vi "MergeMatchPoly.vi"(10 "Poly2D_2":T1, 11 "Poly2D_1":T1) -> (2 "Matched":bool, 3 "Poly2D":T1)   [LabVIEW 2014]
uses:
  TypeDefs/Poly2D.ctl
  TypeDefs/Point2D.ctl
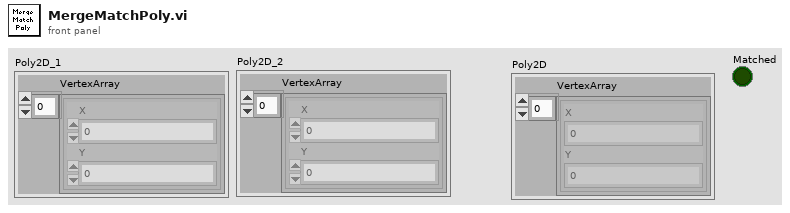
[diagram p1: front panel]
types:
  T1 = typedef "Poly2D.ctl" = cluster{"VertexArray":T2[]}
  T2 = typedef "Point2D.ctl" = cluster{"X":sgl, "Y":sgl}
  T3 = enum16{"V1V1", "V1V2", "V2V1", "V2V2", "NoMatch"}
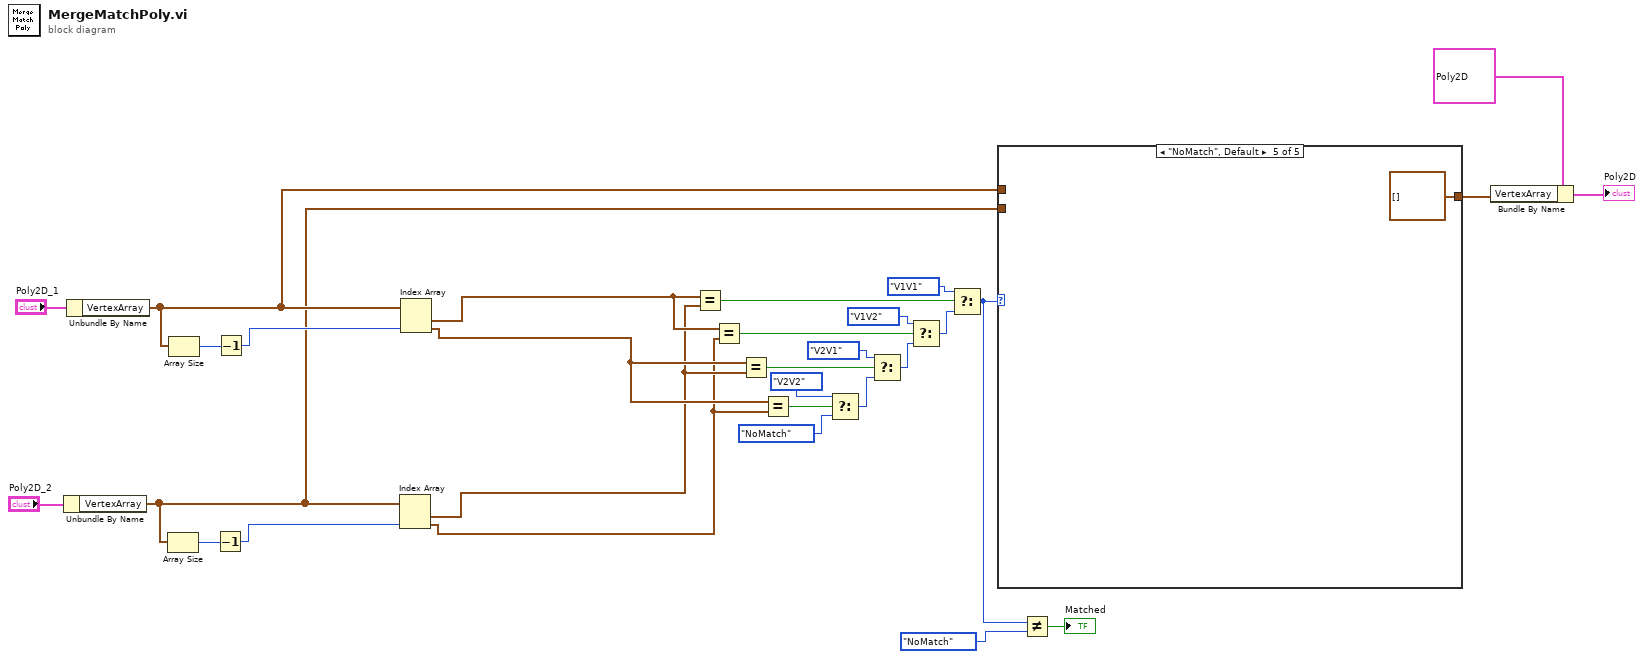
[diagram p0: block diagram]
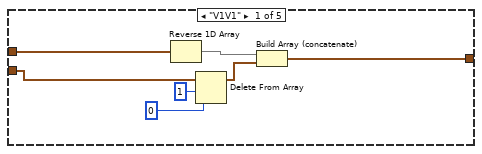
[diagram p2: hidden frame]
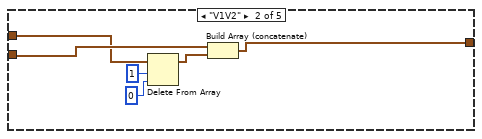
[diagram p3: hidden frame]
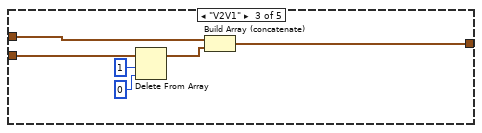
[diagram p4: hidden frame]
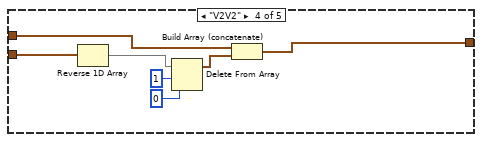
[diagram p5: hidden frame]
diagram:
  n1 = Unbundle By Name("Poly2D_2") -> ("VertexArray"=w4:T2[])
  n2 = Unbundle By Name("Poly2D_1") -> ("VertexArray"=w6:T2[])
  n3 = Array Size(array=w4) -> (size(s)=w27:i32)
  n4 = Array Size(array=w6) -> (size(s)=w30:i32)
  n5 = Decrement(x=w27) -> (x-1=w28:i32)
  n6 = Decrement(x=w30) -> (x-1=w29:i32)
  n7 = Index Array(array=w4, index #2=w28) -> (element #1=w9:T2, element #2=w8:T2)  [unwired: 1 in]
  n8 = Index Array(array=w6, index #2=w29) -> (element #1=w11:T2, element #2=w10:T2)  [unwired: 1 in]
  n9 = Equal?(x=w11, y=w9) -> (x = y?=w26:bool)
  n10 = Equal?(x=w11, y=w8) -> (x = y?=w24:bool)
  n11 = Equal?(x=w10, y=w9) -> (x = y?=w23:bool)
  n12 = Equal?(x=w10, y=w8) -> (x = y?=w21:bool)
  n13 = Select(t=T3."V2V2" ("f"), s=w21, f=T3."NoMatch") -> (s? t:f=w20:T3)
  n14 = Select(t=T3."V2V1" ("f"), s=w23, f=w20) -> (s? t:f=w22:T3)
  n15 = Select(t=T3."V1V2" ("f"), s=w24, f=w22) -> (s? t:f=w25:T3)
  n16 = Select(t=T3."V1V1" ("f"), s=w26, f=w25) -> (s? t:f=w14:T3)
  n17 = case shown="\"NoMatch\", Default" w14 {
    tunnel: w6 -> [w37 w41 w49 w55 _]
    tunnel: w4 -> [w33 w42 w47 w56 _]
    tunnel: [w35 w43 w48 w54 T2[] []] -> w2
    frame "V1V1" {
      n18 = Reverse 1D Array(array=w37) -> (reversed array=w36:T2[])
      n19 = Delete From Array(array=w33, length=1, index=0) -> (array with subset deleted=w32:T2[])  [unwired: 1 out]
      n20 = Build Array (concatenate)(w36, w32) -> (w35:T2[])
    }
    frame "V1V2" {
      n21 = Delete From Array(array=w41, length=1, index=0) -> (array with subset deleted=w38:T2[])  [unwired: 1 out]
      n22 = Build Array (concatenate)(w42, w38) -> (w43:T2[])
    }
    frame "V2V1" {
      n23 = Delete From Array(array=w47, length=1, index=0) -> (array with subset deleted=w44:T2[])  [unwired: 1 out]
      n24 = Build Array (concatenate)(w49, w44) -> (w48:T2[])
    }
    frame "V2V2" {
      n25 = Reverse 1D Array(array=w56) -> (reversed array=w53:T2[])
      n26 = Delete From Array(array=w53, length=1, index=0) -> (array with subset deleted=w52:T2[])  [unwired: 1 out]
      n27 = Build Array (concatenate)(w55, w52) -> (w54:T2[])
    }
    frame "NoMatch", Default {
    }
  }
  n28 = Not Equal?(x=w14, y=T3."NoMatch") -> (x != y?=→"Matched":bool)
  n29 = Bundle By Name(cluster=T1 {"VertexArray"=[{"X"=8.830601, "Y"=7.172068}, {"X"=9.048535, "Y"=7.0468507}, {"X"=7.186762, "Y"=7.89218}, {"X"=7.186762, "Y"=7.89218}, {"X"=7.7402935, "Y"=7.713683}, {"X"=8.830601, "Y"=7.172068}, {"X"=8.385021, "Y"=7.4258633}, {"X"=7.7402935, "Y"=7.713683}, {"X"=9.932331, "Y"=6.418683}, {"X"=9.839655, "Y"=6.4924364}, {"X"=9.9016285, "Y"=6.443779}, {"X"=9.598942, "Y"=6.669884}, {"X"=9.440515, "Y"=6.776763}, {"X"=9.048535, "Y"=7.0468507}, {"X"=8.263897, "Y"=7.4805827}, {"X"=8.113029, "Y"=7.547746}, {"X"=8.385021, "Y"=7.4258633}, {"X"=-0.8597107, "Y"=6.3534126}, {"X"=-0.7344762, "Y"=6.2797923}, {"X"=-1.3683765, "Y"=6.656569}, {"X"=-1.5755129, "Y"=6.777237}, {"X"=-1.9615697, "Y"=6.9872913}, {"X"=-0.86309165, "Y"=6.3554897}, {"X"=0.7361049, "Y"=6.279792}, {"X"=0.7496544, "Y"=6.2877717}, {"X"=0.88590366, "Y"=6.367886}, {"X"=1.1839321, "Y"=6.5489907}, {"X"=1.7457985, "Y"=6.866745}, {"X"=1.6707515, "Y"=6.8289485}, {"X"=1.5142502, "Y"=6.7378664}, {"X"=1.5142502, "Y"=6.7378664}, {"X"=1.1839321, "Y"=6.5489907}, {"X"=0.88590366, "Y"=6.367886}, {"X"=0.8825039, "Y"=6.3658695}, {"X"=-9.596155, "Y"=6.670636}, {"X"=-9.82825, "Y"=6.4999356}, {"X"=-9.82825, "Y"=6.4999356}, {"X"=-9.930481, "Y"=6.418602}, {"X"=-8.38339, "Y"=7.4258623}, {"X"=-9.046905, "Y"=7.0468526}, {"X"=-9.439066, "Y"=6.7766366}, {"X"=-7.7386646, "Y"=7.7136784}, {"X"=-8.38339, "Y"=7.4258623}, {"X"=-7.185123, "Y"=7.89218}, {"X"=-7.439444, "Y"=7.8096337}, {"X"=-7.2370896, "Y"=7.874528}, {"X"=-7.113704, "Y"=7.913477}, {"X"=-7.6962314, "Y"=7.727286}, {"X"=5.3867097, "Y"=8.087741}, {"X"=5.732113, "Y"=8.092253}, {"X"=5.9348326, "Y"=8.090443}, {"X"=6.061366, "Y"=8.076636}, {"X"=6.061366, "Y"=8.076636}, {"X"=2.5593295, "Y"=7.295466}, {"X"=2.7117634, "Y"=7.365449}, {"X"=3.1518545, "Y"=7.5595336}, {"X"=3.387326, "Y"=7.651701}, {"X"=3.6230888, "Y"=7.737315}, {"X"=3.6230888, "Y"=7.737315}, {"X"=4.127137, "Y"=7.8904243}, {"X"=4.6575503, "Y"=8.007021}, {"X"=5.21036, "Y"=8.077528}, {"X"=4.851308, "Y"=8.034141}, {"X"=3.8247945, "Y"=7.7963767}, {"X"=4.3288827, "Y"=7.9346447}, {"X"=6.589266, "Y"=8.020231}, {"X"=6.589266, "Y"=8.020231}, {"X"=7.0844173, "Y"=7.9209275}, {"X"=7.1052027, "Y"=7.9160075}, {"X"=7.1153355, "Y"=7.9134755}, {"X"=11.066484, "Y"=5.9259615}, {"X"=11.296258, "Y"=5.921032}, {"X"=10.557279, "Y"=6.071126}, {"X"=10.38447, "Y"=6.147894}, {"X"=10.217855, "Y"=6.2337523}, {"X"=10.063343, "Y"=6.3245797}, {"X"=9.958954, "Y"=6.399936}, {"X"=11.366602, "Y"=6.3154464}, {"X"=11.3581505, "Y"=6.325527}, {"X"=11.381495, "Y"=5.947889}, {"X"=11.051102, "Y"=5.927362}, {"X"=11.428065, "Y"=6.2203074}, {"X"=11.366602, "Y"=6.3154464}, {"X"=11.4614525, "Y"=6.1327662}, {"X"=11.428065, "Y"=6.2203074}, {"X"=11.465086, "Y"=6.056186}, {"X"=11.4614525, "Y"=6.1327662}, {"X"=11.438299, "Y"=5.9936595}, {"X"=11.465086, "Y"=6.056186}, {"X"=11.438299, "Y"=5.9936595}, {"X"=11.354124, "Y"=5.938431}, {"X"=11.296258, "Y"=5.921032}, {"X"=11.185439, "Y"=5.914531}, {"X"=11.114248, "Y"=5.9222054}, {"X"=10.897281, "Y"=5.9582825}, {"X"=10.843447, "Y"=5.9742303}, {"X"=10.732583, "Y"=6.0081234}, {"X"=11.066484, "Y"=5.9259615}, {"X"=10.732583, "Y"=6.0081234}, {"X"=10.719951, "Y"=6.0130906}, {"X"=10.728581, "Y"=6.0096717}, {"X"=10.450941, "Y"=6.118535}, {"X"=10.289857, "Y"=6.1987867}, {"X"=10.174761, "Y"=6.259248}, {"X"=-0.3831223, "Y"=6.131223}, {"X"=-0.06600832, "Y"=6.079455}, {"X"=0.7361049, "Y"=6.279792}, {"X"=0.49233958, "Y"=6.1676245}, {"X"=0.41289893, "Y"=6.1388397}, {"X"=0.34931928, "Y"=6.1239376}, {"X"=0.06932907, "Y"=6.079732}, {"X"=0.06932907, "Y"=6.079732}, {"X"=-0.3457704, "Y"=6.1236205}, {"X"=-0.7011162, "Y"=6.2621675}, {"X"=-0.3831223, "Y"=6.131223}, {"X"=-0.7344762, "Y"=6.2797923}, {"X"=0.020335363, "Y"=6.074264}, {"X"=-2.5576975, "Y"=7.295468}, {"X"=-2.4127276, "Y"=7.2203803}, {"X"=-2.034087, "Y"=7.027823}, {"X"=-2.5576975, "Y"=7.295468}, {"X"=-2.9499915, "Y"=7.4758196}, {"X"=-2.7095613, "Y"=7.3651953}, {"X"=-5.784939, "Y"=8.094156}, {"X"=-5.5782948, "Y"=8.096169}, {"X"=-5.3852587, "Y"=8.087761}, {"X"=-5.208071, "Y"=8.077488}, {"X"=-5.208071, "Y"=8.077488}, {"X"=-3.3850975, "Y"=7.6514883}, {"X"=-3.150348, "Y"=7.5595837}, {"X"=-3.8916922, "Y"=7.821445}, {"X"=-3.6214588, "Y"=7.73732}, {"X"=-4.6554594, "Y"=8.006941}, {"X"=-4.327599, "Y"=7.934705}, {"X"=-4.1253557, "Y"=7.890371}, {"X"=-6.50035, "Y"=8.036642}, {"X"=-6.0605617, "Y"=8.076551}, {"X"=-5.933233, "Y"=8.090459}, {"X"=-7.0827866, "Y"=7.9209275}, {"X"=-6.5884337, "Y"=8.020078}, {"X"=-7.103572, "Y"=7.916008}, {"X"=-7.103572, "Y"=7.916008}, {"X"=1.9629927, "Y"=6.9872847}, {"X"=2.0286674, "Y"=7.024026}, {"X"=2.3005672, "Y"=7.166774}, {"X"=2.4886727, "Y"=7.2611537}, {"X"=2.5593295, "Y"=7.295466}, {"X"=2.2341883, "Y"=7.1319356}, {"X"=-11.046527, "Y"=5.9253874}, {"X"=-11.183571, "Y"=5.914618}, {"X"=-11.287836, "Y"=5.9220977}, {"X"=-10.211346, "Y"=6.231735}, {"X"=-10.551163, "Y"=6.075544}, {"X"=-10.033587, "Y"=6.345599}, {"X"=-10.211346, "Y"=6.231735}, {"X"=-10.033587, "Y"=6.345599}, {"X"=-10.060636, "Y"=6.324052}, {"X"=-11.438604, "Y"=5.9953485}, {"X"=-11.465441, "Y"=6.0578756}, {"X"=-11.428589, "Y"=6.222046}, {"X"=-11.369982, "Y"=6.305766}, {"X"=-11.363838, "Y"=6.3148956}, {"X"=-11.336758, "Y"=6.3461637}, {"X"=-11.306279, "Y"=5.9260035}, {"X"=-11.38179, "Y"=5.9495883}, {"X"=-11.417481, "Y"=6.239176}, {"X"=-11.363838, "Y"=6.3148956}, {"X"=-11.428589, "Y"=6.222046}, {"X"=-11.461873, "Y"=6.134476}, {"X"=-11.46389, "Y"=6.079863}, {"X"=-11.465441, "Y"=6.0578756}, {"X"=-11.438604, "Y"=5.9953485}, {"X"=-11.38179, "Y"=5.9495883}, {"X"=-11.251305, "Y"=5.9200234}, {"X"=-11.183571, "Y"=5.914618}, {"X"=-11.046527, "Y"=5.9253874}, {"X"=-10.892313, "Y"=5.956102}, {"X"=-10.892313, "Y"=5.956102}, {"X"=-10.557951, "Y"=6.072264}, {"X"=-10.56045, "Y"=6.071302}, {"X"=-10.727159, "Y"=6.0057144}, {"X"=-10.379647, "Y"=6.146689}, {"X"=-10.379647, "Y"=6.146689}, {"X"=10.444521, "Y"=7.162137}, {"X"=10.147654, "Y"=7.396959}, {"X"=11.135348, "Y"=6.5475297}, {"X"=10.8437395, "Y"=6.8065333}, {"X"=11.135348, "Y"=6.5475297}, {"X"=7.7880063, "Y"=8.844079}, {"X"=9.709546, "Y"=7.7424564}, {"X"=9.572357, "Y"=7.8359795}, {"X"=9.48678, "Y"=7.8936634}, {"X"=9.290509, "Y"=8.026892}, {"X"=8.41312, "Y"=8.549493}, {"X"=7.7880063, "Y"=8.844079}, {"X"=10.147654, "Y"=7.396959}, {"X"=8.9828415, "Y"=8.233359}, {"X"=9.290509, "Y"=8.026892}, {"X"=8.2803135, "Y"=8.623675}, {"X"=-10.352315, "Y"=7.234274}, {"X"=-10.44289, "Y"=7.162137}, {"X"=-9.570726, "Y"=7.8359795}, {"X"=-9.707915, "Y"=7.7424564}, {"X"=-10.352315, "Y"=7.234274}, {"X"=-7.7862473, "Y"=8.8441515}, {"X"=-8.180492, "Y"=8.666639}, {"X"=-8.678174, "Y"=8.404416}, {"X"=-8.24564, "Y"=8.638364}, {"X"=-8.278681, "Y"=8.623679}, {"X"=-8.678174, "Y"=8.404416}, {"X"=-9.570726, "Y"=7.8359795}, {"X"=-9.404453, "Y"=7.9493356}, {"X"=-9.108857, "Y"=8.149092}, {"X"=-9.288878, "Y"=8.026892}, {"X"=-11.273474, "Y"=6.4113665}, {"X"=-11.126271, "Y"=6.5544534}, {"X"=-10.842109, "Y"=6.8065333}, {"X"=-10.44289, "Y"=7.162137}, {"X"=-9.838867, "Y"=7.63992}, {"X"=-9.838867, "Y"=7.63992}, {"X"=-9.608428, "Y"=7.8105674}, {"X"=2.3092422, "Y"=9.555755}, {"X"=6.897631, "Y"=9.15439}, {"X"=6.9663086, "Y"=9.135237}, {"X"=6.826199, "Y"=9.173445}, {"X"=6.826199, "Y"=9.173445}, {"X"=6.8652363, "Y"=9.162923}, {"X"=7.4247684, "Y"=8.983244}, {"X"=7.478522, "Y"=8.961372}, {"X"=6.9663086, "Y"=9.135237}, {"X"=7.0981107, "Y"=9.089703}, {"X"=-7.0928435, "Y"=9.091241}, {"X"=-7.0928435, "Y"=9.091241}, {"X"=-7.476928, "Y"=8.961346}, {"X"=-7.4378753, "Y"=8.977723}, {"X"=-2.30762, "Y"=9.555743}, {"X"=-6.9646783, "Y"=9.135236}, {"X"=-6.8925557, "Y"=9.155159}, {"X"=6.644459, "Y"=9.217671}, {"X"=4.169504, "Y"=9.464814}, {"X"=3.7893963, "Y"=9.464789}, {"X"=3.404949, "Y"=9.4514675}, {"X"=5.0040536, "Y"=9.452098}, {"X"=3.0630891, "Y"=9.468226}, {"X"=3.0630891, "Y"=9.468226}, {"X"=2.724652, "Y"=9.495395}, {"X"=2.8233345, "Y"=9.493452}, {"X"=5.3548465, "Y"=9.425313}, {"X"=5.700839, "Y"=9.381838}, {"X"=6.4296727, "Y"=9.26174}, {"X"=6.644459, "Y"=9.217671}, {"X"=6.0274963, "Y"=9.334079}, {"X"=6.0274963, "Y"=9.334079}, {"X"=5.7321496, "Y"=9.377271}, {"X"=5.4556003, "Y"=9.414961}, {"X"=5.175468, "Y"=9.441919}, {"X"=4.65047, "Y"=9.461544}, {"X"=5.0040536, "Y"=9.452098}, {"X"=4.65047, "Y"=9.461544}, {"X"=4.607755, "Y"=9.461863}, {"X"=4.169504, "Y"=9.464814}, {"X"=3.7893963, "Y"=9.464789}, {"X"=3.404949, "Y"=9.4514675}, {"X"=-2.5918474, "Y"=9.499708}, {"X"=-2.7230513, "Y"=9.495405}, {"X"=-4.4270477, "Y"=9.454551}, {"X"=-4.618484, "Y"=9.458359}, {"X"=-5.072798, "Y"=9.436931}, {"X"=-6.491574, "Y"=9.240687}, {"X"=-6.7941, "Y"=9.181162}, {"X"=-4.618484, "Y"=9.458359}, {"X"=-3.0264053, "Y"=9.4683485}, {"X"=-3.0264053, "Y"=9.4683485}, {"X"=-3.2801545, "Y"=9.449338}, {"X"=-3.2801545, "Y"=9.449338}, {"X"=-3.5855074, "Y"=9.461267}, {"X"=-3.3309553, "Y"=9.444425}, {"X"=-3.9134116, "Y"=9.468681}, {"X"=-3.6864495, "Y"=9.468745}, {"X"=-4.239195, "Y"=9.465216}, {"X"=-4.1545463, "Y"=9.471141}, {"X"=-6.2067986, "Y"=9.297449}, {"X"=-5.920551, "Y"=9.346562}, {"X"=-5.639876, "Y"=9.383647}, {"X"=-5.3612723, "Y"=9.4128685}, {"X"=-5.0972753, "Y"=9.434096}, {"X"=-4.8120456, "Y"=9.44821}, {"X"=-6.2067986, "Y"=9.297449}, {"X"=-5.920551, "Y"=9.346562}, {"X"=-5.5172114, "Y"=9.401878}, {"X"=-5.8545833, "Y"=9.354088}, {"X"=2.2132256, "Y"=9.58271}, {"X"=1.8189816, "Y"=9.648704}, {"X"=1.8189816, "Y"=9.648704}, {"X"=2.2132256, "Y"=9.58271}, {"X"=-1.6634326, "Y"=9.665585}, {"X"=-1.8177922, "Y"=9.648689}, {"X"=-2.2115984, "Y"=9.582698}, {"X"=-1.9781245, "Y"=9.618462}, {"X"=0.72814083, "Y"=12.73701}, {"X"=-0.4196546, "Y"=12.743518}, {"X"=0.0007652063, "Y"=12.753558}, {"X"=0.5166687, "Y"=12.742718}, {"X"=0.4116929, "Y"=12.74487}, {"X"=1.0176144, "Y"=12.704265}, {"X"=1.4621797, "Y"=10.655392}, {"X"=1.5545752, "Y"=9.940707}, {"X"=1.4498512, "Y"=10.855028}, {"X"=1.4578543, "Y"=10.732892}, {"X"=1.5545752, "Y"=9.940707}, {"X"=1.6384071, "Y"=9.697788}, {"X"=1.6650634, "Y"=9.665521}, {"X"=1.5937715, "Y"=9.786305}, {"X"=1.5833964, "Y"=9.82258}, {"X"=1.4787083, "Y"=10.454523}, {"X"=1.4787083, "Y"=10.454523}, {"X"=1.5225716, "Y"=10.112019}, {"X"=1.5252, "Y"=10.098917}, {"X"=1.5426022, "Y"=10.012731}, {"X"=1.5040516, "Y"=10.237594}, {"X"=1.4989743, "Y"=10.272214}, {"X"=-1.6634326, "Y"=9.665585}, {"X"=-1.6236622, "Y"=9.727999}, {"X"=-1.5983242, "Y"=9.791381}, {"X"=-1.552802, "Y"=9.935697}, {"X"=-1.5983242, "Y"=9.791381}, {"X"=-1.5869727, "Y"=9.816154}, {"X"=-1.587823, "Y"=9.813162}, {"X"=-1.5209501, "Y"=10.100272}, {"X"=-1.4973384, "Y"=10.267358}, {"X"=-1.4585742, "Y"=10.705285}, {"X"=-1.4635025, "Y"=10.629503}, {"X"=-1.4770607, "Y"=10.45756}, {"X"=-1.4482204, "Y"=10.855038}, {"X"=-1.5474311, "Y"=9.963546}, {"X"=-1.4605238, "Y"=10.667121}, {"X"=-1.4973384, "Y"=10.267358}, {"X"=-1.3789781, "Y"=11.701954}, {"X"=-1.329632, "Y"=12.03006}, {"X"=-1.4286721, "Y"=11.182402}, {"X"=-1.0699232, "Y"=12.697788}, {"X"=-1.0901189, "Y"=12.68052}, {"X"=-1.1646048, "Y"=12.571568}, {"X"=-1.2407196, "Y"=12.380032}, {"X"=-1.2720493, "Y"=12.2814455}, {"X"=-1.0159835, "Y"=12.704266}, {"X"=-1.3427985, "Y"=11.95073}, {"X"=-1.4286721, "Y"=11.182402}, {"X"=-1.4014932, "Y"=11.485938}, {"X"=-1.4188328, "Y"=11.319262}, {"X"=-1.2407196, "Y"=12.380032}, {"X"=-1.1646048, "Y"=12.571568}, {"X"=-1.0901189, "Y"=12.68052}, {"X"=1.1517563, "Y"=12.598272}, {"X"=1.04348, "Y"=12.704147}, {"X"=1.0855013, "Y"=12.679428}, {"X"=1.2149384, "Y"=12.468784}, {"X"=1.1729327, "Y"=12.554751}, {"X"=1.1517563, "Y"=12.598272}, {"X"=1.3806208, "Y"=11.686752}, {"X"=1.4204677, "Y"=11.315399}, {"X"=1.4296497, "Y"=11.192336}, {"X"=1.4498512, "Y"=10.855028}, {"X"=1.3312752, "Y"=12.016102}, {"X"=1.3806208, "Y"=11.686752}, {"X"=1.2736847, "Y"=12.293916}, {"X"=1.2751907, "Y"=12.2876835}, {"X"=1.3312752, "Y"=12.016102}, {"X"=1.2740316, "Y"=12.292477}, {"X"=1.2736847, "Y"=12.293916}, {"X"=1.1150376, "Y"=12.643135}, {"X"=-12.02701, "Y"=-8.883595}, {"X"=-11.930874, "Y"=-8.755775}, {"X"=-12.135208, "Y"=-9.147686}, {"X"=-12.100296, "Y"=-9.031299}, {"X"=-12.095111, "Y"=-9.902619}, {"X"=-12.067877, "Y"=-9.970935}, {"X"=-12.029266, "Y"=-10.067103}, {"X"=-12.029266, "Y"=-10.067103}, {"X"=-11.9856825, "Y"=-10.148499}, {"X"=-12.142309, "Y"=-9.728694}, {"X"=-12.127801, "Y"=-9.782524}, {"X"=-12.1486845, "Y"=-9.194613}, {"X"=-12.170822, "Y"=-9.369725}, {"X"=-12.1705885, "Y"=-9.389268}, {"X"=-12.168238, "Y"=-9.549478}, {"X"=-12.168238, "Y"=-9.549478}, {"X"=-11.8144655, "Y"=-8.65208}, {"X"=-11.7577095, "Y"=-8.616993}, {"X"=-11.8144655, "Y"=-8.65208}, {"X"=-12.02701, "Y"=-8.883595}, {"X"=-12.016741, "Y"=-8.869859}, {"X"=-12.135208, "Y"=-9.147686}, {"X"=-11.294352, "Y"=-10.777359}, {"X"=-11.318705, "Y"=-10.768083}, {"X"=-11.894479, "Y"=-10.297557}, {"X"=-11.864539, "Y"=-10.3413925}, {"X"=-11.542754, "Y"=-10.650674}, {"X"=-11.322815, "Y"=-10.765945}, {"X"=-11.660817, "Y"=-10.56013}, {"X"=-11.684228, "Y"=-10.5376215}, {"X"=-11.768559, "Y"=-10.456095}, {"X"=-11.768559, "Y"=-10.456095}, {"X"=-11.318705, "Y"=-10.768083}, {"X"=-11.864539, "Y"=-10.3413925}, {"X"=-11.569865, "Y"=-8.037169}, {"X"=-11.563985, "Y"=-8.070403}, {"X"=-11.552345, "Y"=-8.164364}, {"X"=-11.553843, "Y"=-8.257444}, {"X"=-11.568527, "Y"=-8.345382}, {"X"=-11.595686, "Y"=-8.425903}, {"X"=-11.632769, "Y"=-8.4943}, {"X"=-11.679456, "Y"=-8.552723}, {"X"=-11.734429, "Y"=-8.599825}, {"X"=-11.700265, "Y"=-8.574736}, {"X"=-11.650671, "Y"=-8.521496}, {"X"=-11.61017, "Y"=-8.45847}, {"X"=-11.579652, "Y"=-8.387263}, {"X"=-11.558998, "Y"=-8.305826}, {"X"=-11.550331, "Y"=-8.218866}, {"X"=-11.553987, "Y"=-8.128481}, {"X"=-11.3296585, "Y"=-13.300342}, {"X"=-11.256834, "Y"=-13.179006}, {"X"=-11.151226, "Y"=-13.057631}, {"X"=-11.16577, "Y"=-13.070827}, {"X"=-11.1825075, "Y"=-13.090706}, {"X"=-11.051586, "Y"=-12.9728775}, {"X"=-11.051586, "Y"=-12.9728775}, {"X"=-10.939525, "Y"=-12.903137}, {"X"=-10.939525, "Y"=-12.903137}, {"X"=-10.849801, "Y"=-14.563225}, {"X"=-11.164953, "Y"=-14.337027}, {"X"=-11.067114, "Y"=-14.428592}, {"X"=-11.141206, "Y"=-14.359256}, {"X"=-11.164953, "Y"=-14.337027}, {"X"=-10.933373, "Y"=-14.519123}, {"X"=-10.960547, "Y"=-14.504524}, {"X"=-11.250185, "Y"=-14.232005}, {"X"=-11.421939, "Y"=-13.710416}, {"X"=-11.408769, "Y"=-13.850409}, {"X"=-11.419471, "Y"=-13.73668}, {"X"=-11.421939, "Y"=-13.710416}, {"X"=-11.413157, "Y"=-13.569632}, {"X"=-11.382209, "Y"=-13.431717}, {"X"=-11.387743, "Y"=-13.456368}, {"X"=-11.256834, "Y"=-13.179006}, {"X"=-11.26992, "Y"=-13.200806}, {"X"=-11.321019, "Y"=-14.114156}, {"X"=-11.305685, "Y"=-14.139672}, {"X"=-11.413157, "Y"=-13.569632}, {"X"=-11.402093, "Y"=-13.876914}, {"X"=-11.374592, "Y"=-13.986052}, {"X"=-11.250185, "Y"=-14.232005}, {"X"=-11.913404, "Y"=-6.6864777}, {"X"=-11.797986, "Y"=-7.147725}, {"X"=-12.13859, "Y"=-5.825948}, {"X"=-11.913404, "Y"=-6.6864777}, {"X"=-12.225317, "Y"=-5.519531}, {"X"=-12.225317, "Y"=-5.519531}, {"X"=-11.221693, "Y"=-10.810644}, {"X"=-11.294352, "Y"=-10.777359}, {"X"=-11.030285, "Y"=-10.970268}, {"X"=-11.091174, "Y"=-10.905559}, {"X"=-11.160064, "Y"=-10.849495}, {"X"=-11.152487, "Y"=-10.854256}, {"X"=-10.860488, "Y"=-11.333081}, {"X"=-10.880931, "Y"=-11.255504}, {"X"=-10.892451, "Y"=-11.2184515}, {"X"=-10.922376, "Y"=-11.142319}, {"X"=-10.928037, "Y"=-11.131481}, {"X"=-10.928037, "Y"=-11.131481}, {"X"=-10.970161, "Y"=-11.053841}, {"X"=-11.02817, "Y"=-10.972571}, {"X"=-10.973595, "Y"=-11.048819}, {"X"=-11.028286, "Y"=-10.97244}, {"X"=-11.087512, "Y"=-10.908614}, {"X"=-10.665473, "Y"=-12.46586}, {"X"=-10.664033, "Y"=-12.508651}, {"X"=-10.673386, "Y"=-12.582449}, {"X"=-10.694738, "Y"=-12.653376}, {"X"=-10.72751, "Y"=-12.7196455}, {"X"=-10.768068, "Y"=-12.776132}, {"X"=-10.816997, "Y"=-12.825721}, {"X"=-10.902442, "Y"=-12.882612}, {"X"=-10.916191, "Y"=-12.891214}, {"X"=-10.800756, "Y"=-12.811512}, {"X"=-10.754254, "Y"=-12.759442}, {"X"=-10.716546, "Y"=-12.700924}, {"X"=-10.686941, "Y"=-12.633139}, {"X"=-10.668956, "Y"=-12.561274}, {"X"=-10.663047, "Y"=-12.487158}, {"X"=-10.665473, "Y"=-12.46586}, {"X"=-10.710455, "Y"=-14.615379}, {"X"=-10.849801, "Y"=-14.563225}, {"X"=-10.848216, "Y"=-14.563806}, {"X"=-10.7669525, "Y"=-14.595915}, {"X"=-10.30013, "Y"=-14.642541}, {"X"=-10.446137, "Y"=-14.654243}, {"X"=-10.446137, "Y"=-14.654243}, {"X"=-10.563266, "Y"=-14.646091}, {"X"=-10.469295, "Y"=-14.651767}, {"X"=-9.648653, "Y"=-14.927292}, {"X"=-9.645592, "Y"=-14.928906}, {"X"=-9.606909, "Y"=-14.948134}, {"X"=-9.606909, "Y"=-14.948134}, {"X"=-9.846963, "Y"=-14.788051}, {"X"=-9.851051, "Y"=-14.785206}, {"X"=-9.854066, "Y"=-14.783052}, {"X"=-9.772256, "Y"=-14.849932}, {"X"=-9.772256, "Y"=-14.849932}, {"X"=-9.739692, "Y"=-14.872915}, {"X"=-9.722611, "Y"=-14.884181}, {"X"=-9.722611, "Y"=-14.884181}, {"X"=-9.686776, "Y"=-14.906165}, {"X"=-12.650918, "Y"=-3.9329345}, {"X"=-12.648346, "Y"=-3.8170426}, {"X"=-12.631214, "Y"=-3.735219}, {"X"=-12.623239, "Y"=-3.7092106}, {"X"=-12.623239, "Y"=-3.7092106}, {"X"=-12.62978, "Y"=-4.049288}, {"X"=-12.650918, "Y"=-3.9329345}, {"X"=-12.57752, "Y"=-3.6137216}, {"X"=-12.57752, "Y"=-3.6137216}, {"X"=-12.513479, "Y"=-3.534193}, {"X"=-12.513479, "Y"=-3.534193}, {"X"=-12.433673, "Y"=-3.4738154}, {"X"=-12.433673, "Y"=-3.4738154}, {"X"=-12.357601, "Y"=-3.4377882}, {"X"=-12.340974, "Y"=-3.43551}, {"X"=-3.3543682, "Y"=-1.112888}, {"X"=-3.2291064, "Y"=-0.992266}, {"X"=-2.9242365, "Y"=-0.58080864}, {"X"=-3.0170414, "Y"=-0.7281756}, {"X"=-3.2999249, "Y"=-1.0642368}, {"X"=-3.4399374, "Y"=-1.1873536}, {"X"=-3.0855627, "Y"=-0.82208127}, {"X"=-3.0855627, "Y"=-0.82208127}, {"X"=-10.675578, "Y"=-12.364202}, {"X"=-10.771004, "Y"=-11.824437}, {"X"=-10.784014, "Y"=-11.759393}, {"X"=-10.784014, "Y"=-11.759393}, {"X"=-5.6554403, "Y"=5.9907885}, {"X"=-4.815982, "Y"=7.0489526}, {"X"=-4.849929, "Y"=6.9179187}, {"X"=-5.0451655, "Y"=6.464496}, {"X"=-5.2916584, "Y"=6.1826806}, {"X"=-5.162795, "Y"=6.294174}, {"X"=-5.543999, "Y"=6.0281105}, {"X"=-6.3306594, "Y"=6.0232587}, {"X"=-6.6277933, "Y"=6.1670747}, {"X"=-6.934379, "Y"=6.406201}, {"X"=-6.8160934, "Y"=6.3108954}, {"X"=-6.4554677, "Y"=6.0813403}, {"X"=-6.3306594, "Y"=6.0232587}, {"X"=-6.250035, "Y"=6.003523}, {"X"=-5.8642983, "Y"=5.95157}, {"X"=-5.6554403, "Y"=5.9907885}, {"X"=-5.924631, "Y"=5.951281}, {"X"=-4.849929, "Y"=6.9179187}, {"X"=-5.0451655, "Y"=6.464496}, {"X"=-10.292118, "Y"=-14.642107}, {"X"=-10.171297, "Y"=-14.638529}, {"X"=-10.041175, "Y"=-14.666001}, {"X"=-10.041588, "Y"=-14.665805}, {"X"=-10.162641, "Y"=-14.639628}, {"X"=-10.162641, "Y"=-14.639628}, {"X"=-10.164488, "Y"=-14.639059}, {"X"=-10.166433, "Y"=-14.638672}, {"X"=-9.460867, "Y"=-15.017409}, {"X"=-9.437974, "Y"=-15.031419}, {"X"=-9.437974, "Y"=-15.031419}, {"X"=-9.564893, "Y"=-14.966767}, {"X"=-9.525483, "Y"=-14.983645}, {"X"=-9.505892, "Y"=-14.993372}, {"X"=-9.58607, "Y"=-14.956815}, {"X"=-9.854066, "Y"=-14.783052}, {"X"=-9.884875, "Y"=-14.755914}, {"X"=-9.887594, "Y"=-14.7537775}, {"X"=-9.901564, "Y"=-14.742871}, {"X"=-9.548078, "Y"=-14.973137}, {"X"=-3.9709668, "Y"=0.83104026}, {"X"=-3.793563, "Y"=0.96303296}, {"X"=-3.6569257, "Y"=1.1055839}, {"X"=-3.5894172, "Y"=1.7002168}, {"X"=-6.403721, "Y"=1.1754698}, {"X"=-6.3508883, "Y"=1.1123196}, {"X"=-6.3508883, "Y"=1.1123196}, {"X"=-3.8743422, "Y"=0.89098823}, {"X"=-3.673383, "Y"=1.0765003}, {"X"=-4.5997987, "Y"=2.4074922}, {"X"=-4.870421, "Y"=2.4419749}, {"X"=-5.4179683, "Y"=2.447132}, {"X"=-5.843843, "Y"=2.364739}, {"X"=-6.137103, "Y"=2.2173433}, {"X"=-4.5921416, "Y"=0.6193031}, {"X"=-4.246321, "Y"=0.71311134}, {"X"=-4.470907, "Y"=0.6456365}, {"X"=-5.0984373, "Y"=0.6077611}, {"X"=-5.0984373, "Y"=0.6077611}, {"X"=-4.658153, "Y"=0.60572743}, {"X"=-5.2277637, "Y"=0.60893834}, {"X"=-5.792988, "Y"=0.74757576}, {"X"=-6.1827035, "Y"=0.97466177}, {"X"=-4.0832763, "Y"=0.7651222}, {"X"=-3.5581236, "Y"=1.3308722}, {"X"=-3.5581236, "Y"=1.3308722}, {"X"=-3.562323, "Y"=1.6246175}, {"X"=-6.4372854, "Y"=1.2494335}, {"X"=-6.532556, "Y"=1.6240577}, {"X"=-6.472267, "Y"=1.8649976}, {"X"=-6.358427, "Y"=2.0599158}, {"X"=-3.5492315, "Y"=1.3571573}, {"X"=-6.535462, "Y"=1.4654024}, {"X"=-3.5894172, "Y"=1.7002168}, {"X"=-6.53032, "Y"=1.7503738}, {"X"=-4.0369825, "Y"=2.1945257}, {"X"=-4.0369825, "Y"=2.1945257}, {"X"=-6.137103, "Y"=2.2173433}, {"X"=-6.3882627, "Y"=2.0303822}, {"X"=-4.870421, "Y"=2.4419749}, {"X"=-5.4179683, "Y"=2.447132}, {"X"=-5.843843, "Y"=2.364739}, {"X"=-6.7040663, "Y"=7.639021}, {"X"=-6.676446, "Y"=7.650669}, {"X"=-4.9156322, "Y"=7.482542}, {"X"=-4.855164, "Y"=7.3850617}, {"X"=-4.815982, "Y"=7.0489526}, {"X"=-4.8155766, "Y"=7.1894574}, {"X"=-4.8181634, "Y"=7.2813587}, {"X"=-5.878805, "Y"=7.82959}, {"X"=-5.5302444, "Y"=7.8090086}, {"X"=-5.289001, "Y"=7.740003}, {"X"=-6.215815, "Y"=7.7961473}, {"X"=-5.11955, "Y"=7.66165}, {"X"=-5.0015216, "Y"=7.5747905}, {"X"=-6.215815, "Y"=7.7961473}, {"X"=-5.878805, "Y"=7.82959}, {"X"=-5.5302444, "Y"=7.8090086}, {"X"=-5.289001, "Y"=7.740003}, {"X"=-5.0015216, "Y"=7.5747905}, {"X"=-4.978973, "Y"=7.5499973}, {"X"=-5.11955, "Y"=7.66165}, {"X"=-4.855164, "Y"=7.3850617}, {"X"=-6.8678813, "Y"=7.52537}, {"X"=-6.777728, "Y"=7.5995193}, {"X"=-6.856725, "Y"=7.5351534}, {"X"=-6.8603616, "Y"=7.531958}, {"X"=-6.875995, "Y"=7.5181913}, {"X"=-6.888495, "Y"=7.503174}, {"X"=-6.888495, "Y"=7.503174}, {"X"=-6.818737, "Y"=7.5675063}, {"X"=-6.7040663, "Y"=7.639021}, {"X"=-6.777728, "Y"=7.5995193}, {"X"=-6.84122, "Y"=7.5485497}, {"X"=-6.8429217, "Y"=7.5470734}, {"X"=-6.8310695, "Y"=7.5571713}, {"X"=-6.875995, "Y"=7.5181913}, {"X"=-6.8678813, "Y"=7.52537}, {"X"=-6.818737, "Y"=7.5675063}, {"X"=-6.822014, "Y"=7.5647697}, {"X"=-7.0596285, "Y"=6.551442}, {"X"=-7.091569, "Y"=7.302365}, {"X"=-7.0596285, "Y"=6.551442}, {"X"=-7.1912403, "Y"=6.921647}, {"X"=-7.155486, "Y"=7.136137}, {"X"=-7.200834, "Y"=7.019425}, {"X"=-6.894214, "Y"=7.488816}, {"X"=-7.065946, "Y"=7.3290687}, {"X"=-7.086213, "Y"=7.308606}, {"X"=-7.1912403, "Y"=6.921647}, {"X"=-10.025236, "Y"=-14.673826}, {"X"=-9.951885, "Y"=-14.708637}, {"X"=-9.932256, "Y"=-14.721165}, {"X"=-9.319345, "Y"=-15.105489}, {"X"=-8.93562, "Y"=-15.3406515}, {"X"=-9.265467, "Y"=-15.138879}, {"X"=-9.319345, "Y"=-15.105489}, {"X"=-8.488454, "Y"=-15.60559}, {"X"=-8.50379, "Y"=-15.596214}, {"X"=-8.0269165, "Y"=-15.876325}, {"X"=-7.546262, "Y"=-16.157545}, {"X"=-7.6811376, "Y"=-16.072777}, {"X"=-8.93562, "Y"=-15.3406515}, {"X"=-8.50379, "Y"=-15.596214}, {"X"=-8.488454, "Y"=-15.60559}, {"X"=-7.546262, "Y"=-16.157545}, {"X"=-7.4288588, "Y"=-16.223211}, {"X"=-7.2701726, "Y"=-16.31386}, {"X"=12.028641, "Y"=-8.883595}, {"X"=11.803545, "Y"=-8.642787}, {"X"=11.75934, "Y"=-8.616993}, {"X"=11.932505, "Y"=-8.755775}, {"X"=11.945703, "Y"=-8.773437}, {"X"=12.149438, "Y"=-9.191597}, {"X"=12.150315, "Y"=-9.194613}, {"X"=12.172453, "Y"=-9.369725}, {"X"=12.169868, "Y"=-9.549478}, {"X"=11.987313, "Y"=-10.148499}, {"X"=12.096742, "Y"=-9.902619}, {"X"=12.030897, "Y"=-10.067103}, {"X"=11.987313, "Y"=-10.148499}, {"X"=12.14394, "Y"=-9.728694}, {"X"=11.816096, "Y"=-8.65208}, {"X"=12.028641, "Y"=-8.883595}, {"X"=12.101927, "Y"=-9.031299}, {"X"=12.104113, "Y"=-9.038665}, {"X"=12.136839, "Y"=-9.147686}, {"X"=12.150315, "Y"=-9.194613}, {"X"=12.172453, "Y"=-9.369725}, {"X"=12.169868, "Y"=-9.549478}, {"X"=12.14394, "Y"=-9.728694}, {"X"=12.096742, "Y"=-9.902619}, {"X"=11.571496, "Y"=-8.037169}, {"X"=11.555617, "Y"=-8.128481}, {"X"=11.555617, "Y"=-8.128481}, {"X"=11.551962, "Y"=-8.218866}, {"X"=11.560629, "Y"=-8.305826}, {"X"=11.581283, "Y"=-8.387263}, {"X"=11.611801, "Y"=-8.45847}, {"X"=11.652302, "Y"=-8.521496}, {"X"=11.701896, "Y"=-8.574736}, {"X"=11.73606, "Y"=-8.599825}, {"X"=11.553976, "Y"=-8.164364}, {"X"=11.555473, "Y"=-8.257444}, {"X"=11.570158, "Y"=-8.345382}, {"X"=11.597317, "Y"=-8.425903}, {"X"=11.634399, "Y"=-8.4943}, {"X"=11.681087, "Y"=-8.552723}, {"X"=11.38384, "Y"=-13.431717}, {"X"=11.376223, "Y"=-13.986052}, {"X"=11.32265, "Y"=-14.114156}, {"X"=10.962178, "Y"=-14.504524}, {"X"=11.068745, "Y"=-14.428592}, {"X"=11.166584, "Y"=-14.337027}, {"X"=11.142837, "Y"=-14.359256}, {"X"=10.852696, "Y"=-14.562547}, {"X"=10.906145, "Y"=-14.535062}, {"X"=10.917822, "Y"=-12.891214}, {"X"=10.941155, "Y"=-12.903137}, {"X"=11.053217, "Y"=-12.9728775}, {"X"=11.152857, "Y"=-13.057631}, {"X"=11.241991, "Y"=-13.15944}, {"X"=11.318304, "Y"=-13.278711}, {"X"=11.3744755, "Y"=-13.408314}, {"X"=11.331289, "Y"=-13.300342}, {"X"=10.960146, "Y"=-12.914559}, {"X"=11.414788, "Y"=-13.569632}, {"X"=11.152857, "Y"=-13.057631}, {"X"=11.241991, "Y"=-13.15944}, {"X"=11.258465, "Y"=-13.179006}, {"X"=11.414788, "Y"=-13.569632}, {"X"=11.42357, "Y"=-13.710416}, {"X"=11.42357, "Y"=-13.710416}, {"X"=11.410399, "Y"=-13.850409}, {"X"=11.410399, "Y"=-13.850409}, {"X"=11.376223, "Y"=-13.986052}, {"X"=11.32265, "Y"=-14.114156}, {"X"=11.251816, "Y"=-14.232005}, {"X"=11.251816, "Y"=-14.232005}, {"X"=11.068745, "Y"=-14.428592}, {"X"=10.962178, "Y"=-14.504524}, {"X"=12.108151, "Y"=-5.9460087}, {"X"=11.915035, "Y"=-6.6864777}, {"X"=12.631411, "Y"=-4.049288}, {"X"=12.463001, "Y"=-4.6658015}, {"X"=12.140221, "Y"=-5.825948}, {"X"=12.201659, "Y"=-5.5894847}, {"X"=11.571496, "Y"=-8.037169}, {"X"=11.915035, "Y"=-6.6864777}, {"X"=10.66729, "Y"=-12.416573}, {"X"=10.664678, "Y"=-12.487158}, {"X"=10.664678, "Y"=-12.487158}, {"X"=10.670587, "Y"=-12.561274}, {"X"=10.688572, "Y"=-12.633139}, {"X"=10.718177, "Y"=-12.700924}, {"X"=10.755885, "Y"=-12.759442}, {"X"=10.802387, "Y"=-12.811512}, {"X"=10.85663, "Y"=-12.855927}, {"X"=10.665664, "Y"=-12.508651}, {"X"=10.675016, "Y"=-12.582449}, {"X"=10.696369, "Y"=-12.653376}, {"X"=10.729141, "Y"=-12.7196455}, {"X"=10.769699, "Y"=-12.776132}, {"X"=10.917822, "Y"=-12.891214}, {"X"=10.85663, "Y"=-12.855927}, {"X"=9.587701, "Y"=-14.956815}, {"X"=9.648387, "Y"=-14.928349}, {"X"=9.685769, "Y"=-14.907634}, {"X"=9.685769, "Y"=-14.907634}, {"X"=9.706607, "Y"=-14.895271}, {"X"=9.706607, "Y"=-14.895271}, {"X"=9.7413225, "Y"=-14.872915}, {"X"=9.773887, "Y"=-14.849932}, {"X"=9.789424, "Y"=-14.838251}, {"X"=9.789424, "Y"=-14.838251}, {"X"=9.8475485, "Y"=-14.790401}, {"X"=9.855697, "Y"=-14.783052}, {"X"=12.5287, "Y"=-3.5463154}, {"X"=12.579146, "Y"=-3.6137137}, {"X"=12.590708, "Y"=-3.6321623}, {"X"=12.590708, "Y"=-3.6321623}, {"X"=12.3426285, "Y"=-3.4355154}, {"X"=12.359256, "Y"=-3.4377937}, {"X"=12.359256, "Y"=-3.4377937}, {"X"=12.450331, "Y"=-3.4807534}, {"X"=12.450331, "Y"=-3.4807534}, {"X"=12.632841, "Y"=-3.7352073}, {"X"=12.632841, "Y"=-3.7352073}, {"X"=12.651887, "Y"=-3.8513145}, {"X"=12.651887, "Y"=-3.8513145}, {"X"=12.645298, "Y"=-3.9750311}, {"X"=12.645298, "Y"=-3.9750311}, {"X"=3.0186722, "Y"=-0.7281756}, {"X"=2.9258673, "Y"=-0.58080864}, {"X"=3.2307372, "Y"=-0.992266}, {"X"=3.0871935, "Y"=-0.82208127}, {"X"=3.1662605, "Y"=-0.9221965}, {"X"=3.4415681, "Y"=-1.1873536}, {"X"=3.355999, "Y"=-1.112888}, {"X"=3.2307372, "Y"=-0.992266}, {"X"=10.293746, "Y"=-14.642103}, {"X"=10.043219, "Y"=-14.665805}, {"X"=10.042806, "Y"=-14.666001}, {"X"=10.026867, "Y"=-14.673826}, {"X"=10.168064, "Y"=-14.638672}, {"X"=10.166119, "Y"=-14.639059}, {"X"=10.170087, "Y"=-14.63848}, {"X"=10.170087, "Y"=-14.63848}, {"X"=9.889225, "Y"=-14.7537775}, {"X"=9.886506, "Y"=-14.755914}, {"X"=9.861074, "Y"=-14.778302}, {"X"=9.861074, "Y"=-14.778302}, {"X"=9.566524, "Y"=-14.966767}, {"X"=9.549708, "Y"=-14.973137}, {"X"=9.417389, "Y"=-15.04401}, {"X"=9.439605, "Y"=-15.031419}, {"X"=9.494886, "Y"=-15.000398}, {"X"=9.531347, "Y"=-14.98244}, {"X"=9.507523, "Y"=-14.993372}, {"X"=9.462498, "Y"=-15.017409}, {"X"=4.7655854, "Y"=0.60666454}, {"X"=4.900757, "Y"=2.44138}, {"X"=4.445768, "Y"=2.35025}, {"X"=4.0750275, "Y"=2.213103}, {"X"=4.084907, "Y"=0.7651222}, {"X"=5.326706, "Y"=0.63066685}, {"X"=5.719236, "Y"=0.7264725}, {"X"=5.5209336, "Y"=2.4304006}, {"X"=3.8698528, "Y"=2.0458076}, {"X"=3.6970007, "Y"=1.864326}, {"X"=3.6070752, "Y"=1.2053412}, {"X"=3.7241516, "Y"=1.0319262}, {"X"=3.5714078, "Y"=1.6560217}, {"X"=3.5652642, "Y"=1.6428374}, {"X"=3.5714078, "Y"=1.6560217}, {"X"=3.5508623, "Y"=1.3571573}, {"X"=3.553045, "Y"=1.3868557}, {"X"=6.3881073, "Y"=1.1548297}, {"X"=6.4852514, "Y"=1.3510339}, {"X"=6.5348525, "Y"=1.5920166}, {"X"=6.4325643, "Y"=1.9461969}, {"X"=6.002293, "Y"=0.86890256}, {"X"=6.2358575, "Y"=1.0170529}, {"X"=6.320571, "Y"=2.0987613}, {"X"=5.2293944, "Y"=0.60893834}, {"X"=4.659784, "Y"=0.60572743}, {"X"=4.659784, "Y"=0.60572743}, {"X"=5.7946186, "Y"=0.74757576}, {"X"=5.5763397, "Y"=0.685647}, {"X"=4.084907, "Y"=0.7651222}, {"X"=6.352519, "Y"=1.1123196}, {"X"=6.1843343, "Y"=0.97466177}, {"X"=3.7241516, "Y"=1.0319262}, {"X"=6.4053516, "Y"=1.1754698}, {"X"=6.5370927, "Y"=1.4654024}, {"X"=6.531951, "Y"=1.7503738}, {"X"=3.6970007, "Y"=1.864326}, {"X"=3.8698528, "Y"=2.0458076}, {"X"=4.1120195, "Y"=2.2329714}, {"X"=6.3898935, "Y"=2.0303822}, {"X"=5.740962, "Y"=2.4042594}, {"X"=5.1689224, "Y"=2.4760795}, {"X"=4.445768, "Y"=2.35025}, {"X"=4.6014295, "Y"=2.4074922}, {"X"=4.8172107, "Y"=7.1894627}, {"X"=5.491926, "Y"=7.8015456}, {"X"=5.7070355, "Y"=7.828284}, {"X"=5.966891, "Y"=7.8276443}, {"X"=6.2695904, "Y"=7.7851615}, {"X"=6.6780767, "Y"=7.650669}, {"X"=6.705697, "Y"=7.639021}, {"X"=5.022007, "Y"=7.5899568}, {"X"=4.9459004, "Y"=7.5142617}, {"X"=4.884291, "Y"=7.4300137}, {"X"=4.8388834, "Y"=7.3348093}, {"X"=4.8172107, "Y"=7.1894627}, {"X"=5.3497233, "Y"=7.7608624}, {"X"=5.2258754, "Y"=7.7112513}, {"X"=5.113709, "Y"=7.657008}, {"X"=5.7070355, "Y"=7.828284}, {"X"=5.966891, "Y"=7.8276443}, {"X"=6.2695904, "Y"=7.7851615}, {"X"=5.022007, "Y"=7.5899568}, {"X"=5.121181, "Y"=7.66165}, {"X"=5.0031524, "Y"=7.5747905}, {"X"=5.2258754, "Y"=7.7112513}, {"X"=4.8388834, "Y"=7.3348093}, {"X"=4.884291, "Y"=7.4300137}, {"X"=5.491926, "Y"=7.8015456}, {"X"=5.4493246, "Y"=7.7930207}, {"X"=6.835574, "Y"=7.554695}, {"X"=6.8738914, "Y"=7.5214505}, {"X"=6.824801, "Y"=7.5637803}, {"X"=6.705697, "Y"=7.639021}, {"X"=6.710484, "Y"=7.6377482}, {"X"=6.79099, "Y"=7.591445}, {"X"=6.779359, "Y"=7.5995193}, {"X"=6.895845, "Y"=7.488816}, {"X"=6.8901258, "Y"=7.503174}, {"X"=6.8738914, "Y"=7.5214505}, {"X"=6.8476286, "Y"=7.5443726}, {"X"=6.8445525, "Y"=7.5470734}, {"X"=6.79099, "Y"=7.591445}, {"X"=6.824801, "Y"=7.5637803}, {"X"=6.835574, "Y"=7.554695}, {"X"=6.871907, "Y"=7.523237}, {"X"=6.864228, "Y"=7.5299687}, {"X"=7.067577, "Y"=7.3290687}, {"X"=7.0931997, "Y"=7.302365}, {"X"=7.006349, "Y"=6.472289}, {"X"=7.0611887, "Y"=6.5513105}, {"X"=7.1854534, "Y"=6.8420715}, {"X"=7.2024646, "Y"=7.019425}, {"X"=7.067577, "Y"=7.3290687}, {"X"=7.0931997, "Y"=7.302365}, {"X"=7.175538, "Y"=6.74118}, {"X"=9.953516, "Y"=-14.708637}, {"X"=10.026867, "Y"=-14.673826}, {"X"=9.903194, "Y"=-14.742871}, {"X"=9.417389, "Y"=-15.04401}, {"X"=9.369135, "Y"=-15.07428}, {"X"=8.505421, "Y"=-15.596214}, {"X"=8.491675, "Y"=-15.604596}, {"X"=9.267097, "Y"=-15.138879}, {"X"=9.267097, "Y"=-15.138879}, {"X"=8.937251, "Y"=-15.3406515}, {"X"=8.282294, "Y"=-15.731429}, {"X"=8.050529, "Y"=-15.86282}, {"X"=8.069378, "Y"=-15.8505335}, {"X"=7.6827683, "Y"=-16.072777}, {"X"=7.5478926, "Y"=-16.157545}, {"X"=9.187492, "Y"=-15.184627}, {"X"=8.862729, "Y"=-15.382493}, {"X"=8.282294, "Y"=-15.731429}, {"X"=8.4929, "Y"=-15.603772}, {"X"=7.430489, "Y"=-16.223211}, {"X"=7.5478926, "Y"=-16.157545}, {"X"=7.171605, "Y"=-16.371065}, {"X"=7.171605, "Y"=-16.371065}, {"X"=11.320335, "Y"=-10.768083}, {"X"=11.929371, "Y"=-10.2494545}, {"X"=11.917312, "Y"=-10.265866}, {"X"=11.885427, "Y"=-10.314343}, {"X"=11.885427, "Y"=-10.314343}, {"X"=11.834314, "Y"=-10.379304}, {"X"=11.74231, "Y"=-10.482889}, {"X"=11.640282, "Y"=-10.577035}, {"X"=11.544385, "Y"=-10.650674}, {"X"=11.86617, "Y"=-10.3413925}, {"X"=11.295982, "Y"=-10.777359}, {"X"=11.312095, "Y"=-10.770921}, {"X"=11.640282, "Y"=-10.577035}, {"X"=11.74231, "Y"=-10.482889}, {"X"=11.282086, "Y"=-10.783227}, {"X"=11.213371, "Y"=-10.816897}, {"X"=11.14764, "Y"=-10.85966}, {"X"=11.086128, "Y"=-10.911853}, {"X"=11.295982, "Y"=-10.777359}, {"X"=11.029917, "Y"=-10.97244}, {"X"=10.975225, "Y"=-11.048819}, {"X"=10.929667, "Y"=-11.131481}, {"X"=10.894082, "Y"=-11.2184515}, {"X"=10.870948, "Y"=-11.297758}, {"X"=10.887574, "Y"=-11.235525}, {"X"=11.029917, "Y"=-10.97244}, {"X"=11.0298, "Y"=-10.972571}, {"X"=10.971792, "Y"=-11.053841}, {"X"=10.924006, "Y"=-11.142319}, {"X"=11.086128, "Y"=-10.911853}, {"X"=11.14764, "Y"=-10.85966}, {"X"=11.213371, "Y"=-10.816897}, {"X"=10.301758, "Y"=-14.642538}, {"X"=10.293746, "Y"=-14.642103}, {"X"=10.564897, "Y"=-14.646091}, {"X"=10.851432, "Y"=-14.563225}, {"X"=10.747182, "Y"=-14.602583}, {"X"=10.712086, "Y"=-14.615379}, {"X"=10.564897, "Y"=-14.646091}, {"X"=10.862119, "Y"=-11.333081}, {"X"=10.7726345, "Y"=-11.824437}, {"X"=10.677209, "Y"=-12.364202}, {"X"=10.66729, "Y"=-12.416573}, {"X"=4.963912, "Y"=6.637194}, {"X"=4.8515596, "Y"=6.9179187}, {"X"=4.8176155, "Y"=7.048952}, {"X"=5.0467963, "Y"=6.464496}, {"X"=5.8659306, "Y"=5.9515653}, {"X"=5.8659306, "Y"=5.9515653}, {"X"=5.9262633, "Y"=5.951276}, {"X"=6.33229, "Y"=6.0232587}, {"X"=6.33229, "Y"=6.0232587}, {"X"=6.629424, "Y"=6.1670747}, {"X"=6.629424, "Y"=6.1670747}, {"X"=6.817724, "Y"=6.3108954}, {"X"=7.006349, "Y"=6.472289}, {"X"=5.0467963, "Y"=6.464496}, {"X"=5.164426, "Y"=6.294174}, {"X"=5.293289, "Y"=6.1826806}, {"X"=5.4052844, "Y"=6.1176023}, {"X"=5.54563, "Y"=6.0281105}, {"X"=5.54563, "Y"=6.0281105}, {"X"=5.5747533, "Y"=6.0193143}, {"X"=-4.928284, "Y"=-17.347603}, {"X"=-4.485192, "Y"=-17.473867}, {"X"=-4.0872045, "Y"=-17.574154}, {"X"=-6.636535, "Y"=-16.656498}, {"X"=-6.955111, "Y"=-16.489447}, {"X"=-7.032068, "Y"=-16.445217}, {"X"=-6.440816, "Y"=-16.758366}, {"X"=-6.1145263, "Y"=-16.906958}, {"X"=-6.048642, "Y"=-16.935936}, {"X"=-5.657333, "Y"=-17.094572}, {"X"=-4.8739295, "Y"=-17.364567}, {"X"=-3.6903965, "Y"=-17.662962}, {"X"=-3.2915175, "Y"=-17.736147}, {"X"=-5.265338, "Y"=-17.239439}, {"X"=-6.636535, "Y"=-16.656498}, {"X"=-6.1145263, "Y"=-16.906958}, {"X"=-6.3764787, "Y"=-16.788654}, {"X"=-5.657333, "Y"=-17.094572}, {"X"=-5.531905, "Y"=-17.140982}, {"X"=-5.2347617, "Y"=-17.249676}, {"X"=-4.8739295, "Y"=-17.364567}, {"X"=-4.485192, "Y"=-17.473867}, {"X"=-4.0872045, "Y"=-17.574154}, {"X"=-3.6903965, "Y"=-17.662962}, {"X"=3.6075315, "Y"=-17.680258}, {"X"=6.638166, "Y"=-16.656498}, {"X"=6.781946, "Y"=-16.580774}, {"X"=6.956742, "Y"=-16.489447}, {"X"=6.781946, "Y"=-16.580774}, {"X"=3.6075315, "Y"=-17.680258}, {"X"=3.7670631, "Y"=-17.646334}, {"X"=6.2929645, "Y"=-16.828487}, {"X"=5.9106174, "Y"=-16.992453}, {"X"=5.3245015, "Y"=-17.21816}, {"X"=5.133149, "Y"=-17.284317}, {"X"=4.7839193, "Y"=-17.390415}, {"X"=3.6920273, "Y"=-17.662962}, {"X"=6.2929645, "Y"=-16.828487}, {"X"=6.050273, "Y"=-16.935936}, {"X"=5.6589637, "Y"=-17.094572}, {"X"=5.2669687, "Y"=-17.239439}, {"X"=4.8755603, "Y"=-17.364567}, {"X"=4.4868226, "Y"=-17.473867}, {"X"=4.298019, "Y"=-17.521143}, {"X"=-10.260574, "Y"=-3.3069108}, {"X"=-11.283855, "Y"=-3.3711903}, {"X"=-9.970092, "Y"=-3.2923765}, {"X"=-3.4399374, "Y"=-1.1873536}, {"X"=-3.521916, "Y"=-1.2533891}, {"X"=-3.7573729, "Y"=-1.434901}, {"X"=-3.7573729, "Y"=-1.434901}, {"X"=-4.0478854, "Y"=-1.6355752}, {"X"=-4.3772445, "Y"=-1.8462685}, {"X"=-5.34146, "Y"=-2.3618393}, {"X"=-5.662619, "Y"=-2.4989357}, {"X"=-5.024132, "Y"=-2.209944}, {"X"=-4.7063894, "Y"=-2.058018}, {"X"=-4.711721, "Y"=-2.061136}, {"X"=-6.1184225, "Y"=-2.6457238}, {"X"=-6.607805, "Y"=-2.8040211}, {"X"=-12.232183, "Y"=-3.4180868}, {"X"=-12.128426, "Y"=-3.4163973}, {"X"=-12.232183, "Y"=-3.4180868}, {"X"=-8.707709, "Y"=-3.1807067}, {"X"=-9.8188925, "Y"=-3.2787843}, {"X"=-9.738416, "Y"=-3.2713087}, {"X"=-9.06884, "Y"=-3.2148187}, {"X"=-8.707709, "Y"=-3.1807067}, {"X"=-7.530573, "Y"=-3.0147233}, {"X"=-11.738921, "Y"=-3.3929737}, {"X"=-11.843679, "Y"=-3.4006338}, {"X"=-11.843679, "Y"=-3.4006338}, {"X"=-10.702967, "Y"=-3.3331478}, {"X"=-11.072473, "Y"=-3.354675}, {"X"=-11.1448, "Y"=-3.3608747}, {"X"=-10.260574, "Y"=-3.3069108}, {"X"=-11.283855, "Y"=-3.3711903}, {"X"=-9.380922, "Y"=-3.240731}, {"X"=-6.607805, "Y"=-2.8040211}, {"X"=-8.248184, "Y"=-3.1152034}, {"X"=-7.7203517, "Y"=-3.047589}, {"X"=-7.119101, "Y"=-2.9200442}, {"X"=-5.662619, "Y"=-2.4989357}, {"X"=-6.1184225, "Y"=-2.6457238}, {"X"=-5.34146, "Y"=-2.3618393}, {"X"=-5.221523, "Y"=-2.3109796}, {"X"=-4.0478854, "Y"=-1.6355752}, {"X"=-4.3772445, "Y"=-1.8462685}, {"X"=12.233814, "Y"=-3.4180868}, {"X"=12.130056, "Y"=-3.4163973}, {"X"=11.893608, "Y"=-3.404276}, {"X"=11.84531, "Y"=-3.4006338}, {"X"=9.479367, "Y"=-3.2494392}, {"X"=11.740552, "Y"=-3.3929737}, {"X"=7.7219825, "Y"=-3.047589}, {"X"=5.7348065, "Y"=-2.5273833}, {"X"=4.692581, "Y"=-2.0487688}, {"X"=5.2231536, "Y"=-2.3109796}, {"X"=4.7049255, "Y"=-2.056361}, {"X"=4.692581, "Y"=-2.0487688}, {"X"=3.7590036, "Y"=-1.434901}, {"X"=3.6075091, "Y"=-1.3226423}, {"X"=3.6075091, "Y"=-1.3226423}, {"X"=3.4415681, "Y"=-1.1873536}, {"X"=5.7348065, "Y"=-2.5273833}, {"X"=10.849632, "Y"=-3.3406618}, {"X"=11.84531, "Y"=-3.4006338}, {"X"=11.285486, "Y"=-3.3711903}, {"X"=10.407241, "Y"=-3.3139515}, {"X"=9.7400465, "Y"=-3.2713087}, {"X"=9.479367, "Y"=-3.2494392}, {"X"=10.407241, "Y"=-3.3139515}, {"X"=8.70934, "Y"=-3.1807067}, {"X"=7.7219825, "Y"=-3.047589}, {"X"=7.5322037, "Y"=-3.0147233}, {"X"=6.7377086, "Y"=-2.841617}, {"X"=5.2231536, "Y"=-2.3109796}, {"X"=4.173215, "Y"=-1.7233979}, {"X"=2.092016, "Y"=-17.90657}, {"X"=0.42150292, "Y"=-18.00863}, {"X"=0.34319338, "Y"=-18.009645}, {"X"=1.695347, "Y"=-17.944841}, {"X"=3.1908336, "Y"=-17.753933}, {"X"=2.9825726, "Y"=-17.7882}, {"X"=2.7701542, "Y"=-17.82051}, {"X"=2.5594132, "Y"=-17.850025}, {"X"=2.490218, "Y"=-17.859251}, {"X"=3.2931483, "Y"=-17.736147}, {"X"=2.0012887, "Y"=-17.915014}, {"X"=2.0012887, "Y"=-17.915014}, {"X"=0.84556794, "Y"=-17.997324}, {"X"=0.44709656, "Y"=-18.008022}, {"X"=0.42150292, "Y"=-18.00863}, {"X"=1.3231481, "Y"=-17.972385}, {"X"=1.2700415, "Y"=-17.976114}, {"X"=2.690039, "Y"=-17.832129}, {"X"=2.7701542, "Y"=-17.82051}, {"X"=3.0914207, "Y"=-17.77078}, {"X"=0.0008154644, "Y"=-18.009115}, {"X"=-0.0014298288, "Y"=-18.008503}, {"X"=0.0037170372, "Y"=-18.006178}, {"X"=0.0030606594, "Y"=-18.008503}, {"X"=-2.0903852, "Y"=-17.90657}, {"X"=-3.2915175, "Y"=-17.736147}, {"X"=-3.1892028, "Y"=-17.753933}, {"X"=-2.9965718, "Y"=-17.78538}, {"X"=-2.8064823, "Y"=-17.814571}, {"X"=-2.616186, "Y"=-17.841745}, {"X"=-2.3674042, "Y"=-17.87328}, {"X"=-2.4885871, "Y"=-17.859251}, {"X"=-0.0020862846, "Y"=-18.006178}, {"X"=-0.07978936, "Y"=-18.006723}, {"X"=-0.34159136, "Y"=-18.009645}, {"X"=-0.8106943, "Y"=-17.998108}, {"X"=-1.2199664, "Y"=-17.978369}, {"X"=-1.6231827, "Y"=-17.949776}, {"X"=-1.6937162, "Y"=-17.944841}, {"X"=-1.6231827, "Y"=-17.949776}, {"X"=-2.616186, "Y"=-17.841745}, {"X"=-2.8064823, "Y"=-17.814571}, {"X"=-3.0897899, "Y"=-17.77078}, {"X"=-1.2199664, "Y"=-17.978369}, {"X"=-0.8106943, "Y"=-17.998108}, {"X"=-0.00854867, "Y"=3.7263947}, {"X"=-0.0066404296, "Y"=3.7263823}, {"X"=0.008271213, "Y"=3.7263823}, {"X"=-0.76231277, "Y"=2.8479533}, {"X"=0.6740086, "Y"=2.847094}, {"X"=0.6740086, "Y"=2.847094}, {"X"=0.47253898, "Y"=2.847094}, {"X"=-0.07608838, "Y"=3.7179072}, {"X"=-0.4628392, "Y"=3.5587547}, {"X"=-0.3386752, "Y"=3.6528666}, {"X"=-0.07608838, "Y"=3.7179072}, {"X"=0.29774323, "Y"=3.670729}, {"X"=0.34028584, "Y"=3.6528666}, {"X"=0.46445665, "Y"=3.5587547}, {"X"=0.060030755, "Y"=3.720132}, {"X"=0.0101794535, "Y"=3.7263947}, {"X"=-0.4628392, "Y"=3.5587547}, {"X"=-0.49247614, "Y"=3.5338767}, {"X"=-0.49247614, "Y"=3.5338767}, {"X"=-0.48612607, "Y"=3.5097697}, {"X"=-0.45324963, "Y"=3.4870713}, {"X"=-0.39212748, "Y"=3.466576}, {"X"=-0.49027306, "Y"=3.5230303}, {"X"=-0.47441077, "Y"=3.5007813}, {"X"=-0.4386713, "Y"=3.4815457}, {"X"=-0.3861084, "Y"=3.465226}, {"X"=-0.24353056, "Y"=3.4534297}, {"X"=-0.36558542, "Y"=3.4612727}, {"X"=0.010381071, "Y"=3.4437823}, {"X"=-0.008876924, "Y"=3.4437895}, {"X"=-0.008750289, "Y"=3.4437823}, {"X"=0.010381071, "Y"=3.4437823}, {"X"=0.48574132, "Y"=3.544352}, {"X"=0.46445665, "Y"=3.5587547}, {"X"=0.4877475, "Y"=3.5097704}, {"X"=0.49189267, "Y"=3.5230253}, {"X"=0.49409693, "Y"=3.5338771}, {"X"=0.45487154, "Y"=3.4870725}, {"X"=0.4760247, "Y"=3.5007768}, {"X"=0.39375165, "Y"=3.466578}, {"X"=0.44027802, "Y"=3.4815414}, {"X"=0.24528153, "Y"=3.4534278}, {"X"=0.38770628, "Y"=3.465222}, {"X"=0.0105077075, "Y"=3.4437895}, {"X"=1.067618, "Y"=2.7614944}, {"X"=1.0173168, "Y"=2.8046827}, {"X"=1.0106434, "Y"=2.8081396}, {"X"=0.998331, "Y"=2.8126178}, {"X"=0.96865463, "Y"=2.8240356}, {"X"=0.96865463, "Y"=2.8240356}, {"X"=1.0473349, "Y"=2.7850795}, {"X"=1.0565383, "Y"=2.7741954}, {"X"=0.92898184, "Y"=2.8333485}, {"X"=0.92898184, "Y"=2.8333485}, {"X"=0.8959438, "Y"=2.8382154}, {"X"=0.8375098, "Y"=2.8446708}, {"X"=0.88944787, "Y"=2.8387268}, {"X"=0.7639368, "Y"=2.8479538}, {"X"=-1.045704, "Y"=2.7850792}, {"X"=-1.0445257, "Y"=2.7859926}, {"X"=-1.045704, "Y"=2.7850792}, {"X"=-1.0090119, "Y"=2.8081396}, {"X"=-0.9670265, "Y"=2.8240356}, {"X"=-0.8358763, "Y"=2.8446715}, {"X"=-0.7951621, "Y"=2.8454816}, {"X"=-0.7951621, "Y"=2.8454816}, {"X"=-0.8943183, "Y"=2.8382156}, {"X"=-0.8982203, "Y"=2.8373964}, {"X"=-0.8982203, "Y"=2.8373964}, {"X"=-0.9967021, "Y"=2.812618}, {"X"=-1.0090119, "Y"=2.8081396}, {"X"=-1.0659869, "Y"=2.7614949}, {"X"=-1.0549076, "Y"=2.7741952}, {"X"=-0.48852873, "Y"=2.3884056}, {"X"=-0.07730713, "Y"=2.3884056}, {"X"=0.7514543, "Y"=2.386611}, {"X"=-0.07730713, "Y"=2.3884056}, {"X"=-1.14167, "Y"=2.3826506}, {"X"=1.1432979, "Y"=2.3826497}, {"X"=-0.41324222, "Y"=2.0111115}, {"X"=-0.70813435, "Y"=2.0103872}, {"X"=-0.49057758, "Y"=2.0111115}, {"X"=0.70983547, "Y"=2.0103867}, {"X"=0.70983547, "Y"=2.0103867}, {"X"=-0.41324222, "Y"=2.0111115}, {"X"=1.2337487, "Y"=2.4588747}, {"X"=1.2165025, "Y"=2.404758}, {"X"=1.1983142, "Y"=2.397272}, {"X"=1.1722122, "Y"=2.3927495}, {"X"=1.1916199, "Y"=2.3954153}, {"X"=1.1432979, "Y"=2.3826497}, {"X"=1.2353605, "Y"=2.4271605}, {"X"=1.228462, "Y"=2.4146354}, {"X"=1.222558, "Y"=2.4088516}, {"X"=1.2165025, "Y"=2.404758}, {"X"=1.226176, "Y"=2.4763017}, {"X"=1.2289872, "Y"=2.4697802}, {"X"=1.2092305, "Y"=2.4009252}, {"X"=1.2353605, "Y"=2.4271605}, {"X"=1.2364476, "Y"=2.433267}, {"X"=1.2370933, "Y"=2.441883}, {"X"=1.4738536, "Y"=2.006581}, {"X"=1.4669265, "Y"=2.0087044}, {"X"=1.4593807, "Y"=2.009836}, {"X"=1.4574188, "Y"=2.009671}, {"X"=1.5014237, "Y"=1.9812346}, {"X"=1.4986236, "Y"=1.9855362}, {"X"=1.4926502, "Y"=1.9933399}, {"X"=1.4872434, "Y"=1.9984872}, {"X"=1.4812546, "Y"=2.0027587}, {"X"=1.4748765, "Y"=2.0060189}, {"X"=1.4802402, "Y"=2.0035176}, {"X"=1.4971714, "Y"=1.9878777}, {"X"=1.4920352, "Y"=1.9941158}, {"X"=1.4863943, "Y"=1.9993223}, {"X"=1.4593807, "Y"=2.009836}, {"X"=1.459968, "Y"=2.0097}, {"X"=-1.4576082, "Y"=2.009493}, {"X"=-1.457856, "Y"=2.0095024}, {"X"=-1.457856, "Y"=2.0095024}, {"X"=-1.4649794, "Y"=2.008526}, {"X"=-1.4716955, "Y"=2.0065548}, {"X"=-1.4780617, "Y"=2.0036175}, {"X"=-1.4843178, "Y"=1.9994733}, {"X"=-1.4902166, "Y"=1.9941378}, {"X"=-1.4956957, "Y"=1.9875569}, {"X"=-1.4960741, "Y"=1.986977}, {"X"=-1.4960741, "Y"=1.986977}, {"X"=-1.4579788, "Y"=2.009514}, {"X"=-1.4956957, "Y"=1.9875569}, {"X"=-1.4902166, "Y"=1.9941378}, {"X"=-1.4843178, "Y"=1.9994733}, {"X"=-1.4780617, "Y"=2.0036175}, {"X"=-1.4716955, "Y"=2.0065548}, {"X"=-1.2316467, "Y"=2.459709}, {"X"=-1.1959518, "Y"=2.398109}, {"X"=-1.1960353, "Y"=2.3981266}, {"X"=-1.2158687, "Y"=2.406542}, {"X"=-1.2276436, "Y"=2.4172268}, {"X"=-1.2336802, "Y"=2.4300911}, {"X"=-1.2346641, "Y"=2.4445548}, {"X"=-1.2352839, "Y"=2.442157}, {"X"=-1.1959518, "Y"=2.398109}, {"X"=-1.1648246, "Y"=2.3918023}, {"X"=-1.1706961, "Y"=2.3924835}, {"X"=-1.2245513, "Y"=2.476303}, {"X"=-1.2336527, "Y"=2.4271784}, {"X"=-1.2276436, "Y"=2.4172268}, {"X"=-1.1960255, "Y"=2.398121}, {"X"=-1.2145584, "Y"=2.405078}, {"X"=1.5076458, "Y"=1.9700412}, {"X"=1.78655, "Y"=1.4684}, {"X"=1.78655, "Y"=1.4684}, {"X"=1.8523945, "Y"=1.34997}, {"X"=1.8655576, "Y"=1.3262943}, {"X"=1.8931534, "Y"=1.2766625}, {"X"=1.8931534, "Y"=1.2766625}, {"X"=1.9770744, "Y"=1.1257194}, {"X"=1.9836459, "Y"=1.1138973}, {"X"=2.2579062, "Y"=0.62060535}, {"X"=2.3439512, "Y"=0.4658459}, {"X"=2.4375534, "Y"=0.29749277}, {"X"=2.4375534, "Y"=0.29749277}, {"X"=2.5186753, "Y"=0.151581}, {"X"=2.6968968, "Y"=-0.16897915}, {"X"=2.8735185, "Y"=-0.4866523}, {"X"=2.634508, "Y"=-0.056768816}, {"X"=2.8530045, "Y"=-0.44975382}, {"X"=1.1919955, "Y"=2.5377808}, {"X"=1.1919955, "Y"=2.5377808}, {"X"=1.5014237, "Y"=1.9812346}, {"X"=-1.4998013, "Y"=1.9812322}, {"X"=-1.5060034, "Y"=1.970079}, {"X"=-1.784904, "Y"=1.4684283}, {"X"=-1.857495, "Y"=1.3378601}, {"X"=-1.8507538, "Y"=1.3499885}, {"X"=-1.2245513, "Y"=2.476303}, {"X"=-1.0659869, "Y"=2.7614949}, {"X"=-1.7710594, "Y"=1.4933293}, {"X"=-1.8639268, "Y"=1.3262943}, {"X"=-1.8915226, "Y"=1.2766625}, {"X"=-1.9820136, "Y"=1.113902}, {"X"=-2.1730704, "Y"=0.7702549}, {"X"=-2.2562754, "Y"=0.62060535}, {"X"=-2.4359226, "Y"=0.29749277}, {"X"=-2.632877, "Y"=-0.056768816}, {"X"=-2.8513737, "Y"=-0.44975382}, {"X"=-2.3423204, "Y"=0.4658459}, {"X"=-2.5170445, "Y"=0.151581}, {"X"=-2.695266, "Y"=-0.16897915}, {"X"=-2.8718877, "Y"=-0.4866523}, {"X"=-1.9754436, "Y"=1.1257194}, {"X"=-6.1731024, "Y"=0.80225223}, {"X"=-6.4152503, "Y"=1.0218331}, {"X"=-6.608058, "Y"=1.2818588}, {"X"=-6.6882205, "Y"=1.5042956}, {"X"=-6.6324167, "Y"=1.8278004}, {"X"=-6.4458513, "Y"=2.1040184}, {"X"=-6.1973596, "Y"=2.3407633}, {"X"=-5.523589, "Y"=0.5446353}, {"X"=-5.79826, "Y"=2.4814765}, {"X"=-4.867923, "Y"=0.47854578}, {"X"=-5.3243194, "Y"=2.5744805}, {"X"=-3.50968, "Y"=1.0301466}, {"X"=-3.4327807, "Y"=1.2001191}, {"X"=-3.3941116, "Y"=1.382841}, {"X"=-3.4603047, "Y"=1.7814922}, {"X"=-4.809182, "Y"=0.48575115}, {"X"=-4.405914, "Y"=0.54676175}, {"X"=-4.595913, "Y"=2.5052567}, {"X"=-4.0831995, "Y"=0.6346704}, {"X"=-4.1484256, "Y"=2.3729658}, {"X"=-3.6613507, "Y"=0.885137}, {"X"=-3.85941, "Y"=0.7556109}, {"X"=-4.011697, "Y"=0.66795987}, {"X"=-6.1973596, "Y"=2.3407633}, {"X"=-5.79826, "Y"=2.4814765}, {"X"=-5.3243194, "Y"=2.5744805}, {"X"=-4.595913, "Y"=2.5052567}, {"X"=-6.4458513, "Y"=2.1040184}, {"X"=-3.5067923, "Y"=1.8703905}, {"X"=-3.5067923, "Y"=1.8703905}, {"X"=-6.6324167, "Y"=1.8278004}, {"X"=-3.4603047, "Y"=1.7814922}, {"X"=-6.6882205, "Y"=1.5042956}, {"X"=-3.3941116, "Y"=1.382841}, {"X"=-6.608058, "Y"=1.2818588}, {"X"=-3.4327807, "Y"=1.2001191}, {"X"=-6.4152503, "Y"=1.0218331}, {"X"=-3.50968, "Y"=1.0301466}, {"X"=-3.5353258, "Y"=0.9944994}, {"X"=-6.1731024, "Y"=0.80225223}, {"X"=-3.7040718, "Y"=0.85061496}, {"X"=-5.523589, "Y"=0.5446353}, {"X"=-4.405914, "Y"=0.54676175}, {"X"=-4.809182, "Y"=0.48575115}, {"X"=-4.1103888, "Y"=2.2329714}, {"X"=-4.869828, "Y"=2.4418511}, {"X"=-5.417605, "Y"=2.4471264}, {"X"=-5.843739, "Y"=2.3647609}, {"X"=-3.5717738, "Y"=1.6587385}, {"X"=-5.717605, "Y"=0.7264725}, {"X"=-6.403721, "Y"=1.1754698}, {"X"=-4.0733967, "Y"=2.213103}, {"X"=-4.0369825, "Y"=2.1945257}, {"X"=-3.8689134, "Y"=2.0467944}, {"X"=-3.8689134, "Y"=2.0467944}, {"X"=-3.695971, "Y"=1.8667909}, {"X"=-3.7373013, "Y"=1.9342899}, {"X"=-3.5643377, "Y"=1.6428626}, {"X"=-5.574709, "Y"=0.685647}, {"X"=-3.5498102, "Y"=1.3571969}, {"X"=-3.6723025, "Y"=1.0764607}, {"X"=-4.7639546, "Y"=0.60666454}, {"X"=-3.873783, "Y"=0.89096785}, {"X"=-4.470907, "Y"=0.6456365}, {"X"=-5.7393327, "Y"=2.4042227}, {"X"=-4.869828, "Y"=2.4418511}, {"X"=-5.417605, "Y"=2.4471264}, {"X"=-6.31894, "Y"=2.0987613}, {"X"=-6.31894, "Y"=2.0987613}, {"X"=-3.5643377, "Y"=1.6428626}, {"X"=-6.1827035, "Y"=0.97466177}, {"X"=-6.53032, "Y"=1.7503738}, {"X"=-6.3882627, "Y"=2.0303822}, {"X"=-3.5498102, "Y"=1.3571969}, {"X"=-6.5354886, "Y"=1.4654716}, {"X"=-6.53032, "Y"=1.7503738}, {"X"=-3.6723025, "Y"=1.0764607}, {"X"=-6.2342267, "Y"=1.0170529}, {"X"=-6.1827035, "Y"=0.97466177}, {"X"=-6.483632, "Y"=1.3510634}, {"X"=-3.717171, "Y"=1.0358701}, {"X"=-6.403721, "Y"=1.1754698}, {"X"=-6.3864765, "Y"=1.1548297}, {"X"=-6.0006623, "Y"=0.86890256}, {"X"=-5.574709, "Y"=0.685647}, {"X"=-4.470907, "Y"=0.6456365}, {"X"=-4.7639546, "Y"=0.60666454}, {"X"=-5.325075, "Y"=0.63066685}, {"X"=5.768352, "Y"=2.4869251}, {"X"=6.256812, "Y"=2.3057399}, {"X"=3.3904872, "Y"=1.4368991}, {"X"=6.115471, "Y"=0.7700497}, {"X"=4.9278536, "Y"=2.5646243}, {"X"=6.607655, "Y"=1.9358124}, {"X"=4.4356084, "Y"=2.454596}, {"X"=6.7040563, "Y"=1.5566156}, {"X"=4.024505, "Y"=2.3008115}, {"X"=6.6571274, "Y"=1.3635727}, {"X"=3.8814108, "Y"=2.2197797}, {"X"=6.5468025, "Y"=1.168247}, {"X"=3.4867268, "Y"=1.8398644}, {"X"=6.373358, "Y"=0.9706594}, {"X"=3.418811, "Y"=1.2466412}, {"X"=5.567228, "Y"=0.5589959}, {"X"=3.4960277, "Y"=1.0581442}, {"X"=3.6728444, "Y"=0.8732367}, {"X"=5.017665, "Y"=0.49480686}, {"X"=3.9657695, "Y"=0.6925165}, {"X"=4.5461817, "Y"=0.5221703}, {"X"=6.3164315, "Y"=0.9224521}, {"X"=3.474629, "Y"=1.8224995}, {"X"=3.4075844, "Y"=1.5070968}, {"X"=3.3904872, "Y"=1.4368991}, {"X"=5.517816, "Y"=0.5428311}, {"X"=4.866611, "Y"=0.4799412}, {"X"=5.567228, "Y"=0.5589959}, {"X"=4.210116, "Y"=0.57917607}, {"X"=6.115471, "Y"=0.7700497}, {"X"=6.1346426, "Y"=0.7791764}, {"X"=3.9657695, "Y"=0.6925165}, {"X"=6.373358, "Y"=0.9706594}, {"X"=3.543388, "Y"=0.9885701}, {"X"=6.5468025, "Y"=1.168247}, {"X"=3.4960277, "Y"=1.0581442}, {"X"=6.6571274, "Y"=1.3635727}, {"X"=3.418811, "Y"=1.2466412}, {"X"=6.7040563, "Y"=1.5566156}, {"X"=6.607655, "Y"=1.9358124}, {"X"=3.514335, "Y"=1.8804414}, {"X"=6.111094, "Y"=2.3925397}, {"X"=5.4517217, "Y"=2.575982}, {"X"=4.7988167, "Y"=2.5636787}, {"X"=4.1516795, "Y"=2.3743773}, {"X"=3.8814108, "Y"=2.2197797}, {"X"=3.9731412, "Y"=0.83052903}, {"X"=3.795828, "Y"=0.9617485}, {"X"=3.6591375, "Y"=1.1025287}, {"X"=3.5967474, "Y"=1.7109286}, {"X"=4.601434, "Y"=2.407352}, {"X"=4.247952, "Y"=0.71311134}, {"X"=4.5937724, "Y"=0.6193031}, {"X"=6.360058, "Y"=2.0599158}, {"X"=6.473898, "Y"=1.8649976}, {"X"=6.534187, "Y"=1.6240577}, {"X"=6.438916, "Y"=1.2494335}, {"X"=6.352519, "Y"=1.1123196}, {"X"=6.1843343, "Y"=0.97466177}, {"X"=5.7946186, "Y"=0.74757576}, {"X"=5.7946186, "Y"=0.74757576}, {"X"=6.473898, "Y"=1.8649976}, {"X"=4.8706145, "Y"=2.4416611}, {"X"=5.4187417, "Y"=2.447126}, {"X"=5.100068, "Y"=0.6077611}, {"X"=5.2293944, "Y"=0.60893834}, {"X"=5.5763397, "Y"=0.685647}, {"X"=4.5937724, "Y"=0.6193031}, {"X"=4.247952, "Y"=0.71311134}, {"X"=4.084907, "Y"=0.7651222}, {"X"=3.5614526, "Y"=1.3278108}, {"X"=3.5644014, "Y"=1.6208274}, {"X"=3.8754106, "Y"=0.89096767}, {"X"=6.5370927, "Y"=1.4654024}, {"X"=3.5614526, "Y"=1.3278108}, {"X"=3.6739268, "Y"=1.0764607}, {"X"=3.5514364, "Y"=1.3571784}, {"X"=6.534187, "Y"=1.6240577}, {"X"=3.5967474, "Y"=1.7109286}, {"X"=6.138734, "Y"=2.2173433}, {"X"=5.845225, "Y"=2.3647902}, {"X"=4.0386133, "Y"=2.1945257}, {"X"=4.0386133, "Y"=2.1945257}, {"X"=6.360058, "Y"=2.0599158}, {"X"=6.320571, "Y"=2.0987613}, {"X"=4.8706145, "Y"=2.4416611}, {"X"=5.4187417, "Y"=2.447126}, {"X"=6.0050135, "Y"=2.3015885}]}, "VertexArray"=w2) -> (→"Poly2D":T1)
